vi "Read Agent Public Key Refnum.vi"(8 "error in (no error)":errorcluster, 11 "agent public key":T1) -> (0 "error out":errorcluster, 2 "libssh2_agent_publickey*":u64)   [LabVIEW 2013, in "libssh2.lvlib"]
doc: "Gets the pointer to libssh2_agent_publickey associated with <B>agent public key</B>."
uses:
  libssh2.lvlib
  Agent Public Key Refnum.ctl
  Agent Public Key Refnum Data.ctl
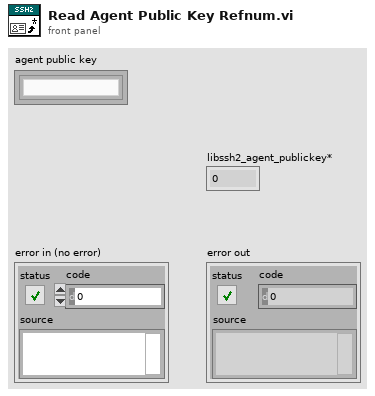
[diagram p1: front panel]
types:
  T1 = typedef "libssh2.lvlib/Agent Public Key Refnum.ctl" = refnum<k1>
  T2 = typedef "libssh2.lvlib/Agent Public Key Refnum Data.ctl" = cluster{"libssh2_agent_publickey*":u64}
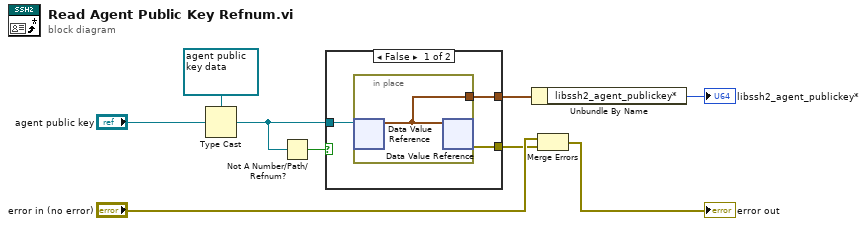
[diagram p0: block diagram]
diagram:
  n1 = Type Cast(type=refnum<data-value> refnum ("data value reference"), x="agent public key") -> (*(type *) &x=w3:refnum<data-value>)
  n2 = Not A Number/Path/Refnum?(number/path/refnum=w3) -> (NaN/Path/Refnum?=w2:bool)
  n3 = case shown="False" w2 {
    tunnel: w3 -> [w12 _]
    tunnel: [w11 _] -> w8
    tunnel: [w10 _] -> w4
    frame False {
      n4 = in-place {
        in-place-border: [w13] -> w11
        n5 = in-place-dvr #1(w12) -> (w13:T2)  [unwired: 1 out]
        n6 = in-place-dvr #1(w13) -> (w10:errorcluster)  [unwired: 1 out]
      }
    }
    frame True {
    }
  }
  n7 = Unbundle By Name(w8) -> ("libssh2_agent_publickey*"=→"libssh2_agent_publickey*":u64)
  n8 = Merge Errors("error in (no error)", w4) -> (→"error out":errorcluster)
